vi "Delete Panel.vi"(8 "error in (no error)":errorcluster caption="错误输入（无错误）", 9 "Abort VI":bool, 10 "SelfNode*":refnum<data-value>) -> (0 "error out":errorcluster caption="错误输出", 2 "BrotherNodeBeDeleted":refnum<data-value>, 3 "ParentNode*":refnum<data-value>)   [LabVIEW 2013, in "PanelDataNode.lvclass"]
uses:
  PanelDataNode.lvclass
  PanelObject/PanelObject.lvclass
  PanelLinkNode/PanelLinkNode.lvclass/PanelLinkNode.ctl
  PanelLinkNode/PanelLinkNode.lvclass
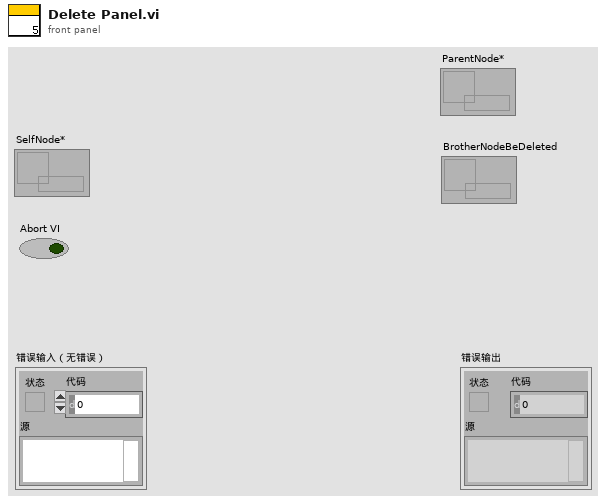
[diagram p1: front panel]
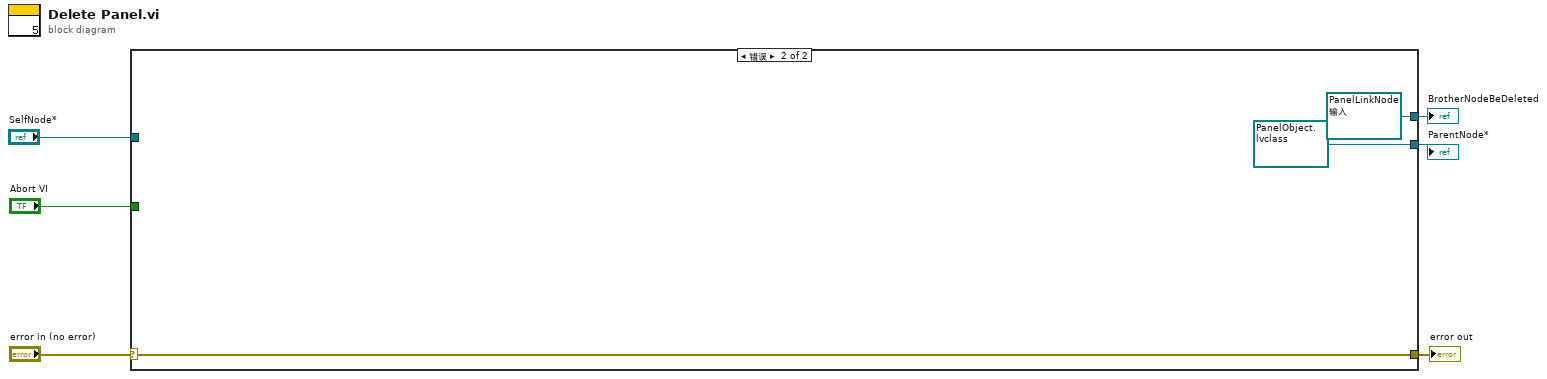
[diagram p0: block diagram]
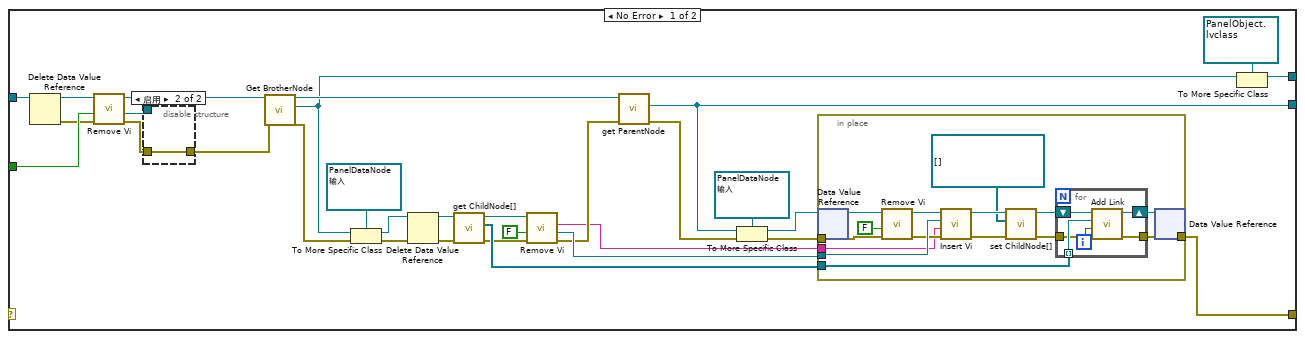
[diagram p2: hidden frame]
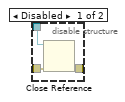
[diagram p3: hidden frame]
diagram:
  n1 = case shown="错误" "error in (no error)" {
    selector: "error in (no error)" -> [_ w65]
    tunnel: [w37 w65] -> w5
    tunnel: "SelfNode*" -> [w16 _]
    tunnel: "Abort VI" -> [w36 _]
    tunnel: [w9 refnum<data-value> refnum ("BrotherNode*")] -> w2
    tunnel: [w7 refnum<data-value> refnum ("ParentNode*")] -> w1
    frame No Error {
      n2 = Delete Data Value Reference(data value reference=w16) -> (data value=w15:refnum<class "PanelDataNode.lvclass">, error out=w14:errorcluster)  [unwired: 1 in]
      n3 = call-dynamic "Remove Vi.vi"("error in"=w14, "Abort VI"=w36, "PanelDataNode 输入"=w15) -> ("error out"=w29:errorcluster, "VI*"=w11:refnum<vi>, "PanelDataNode 输出"=w33:refnum<class "PanelDataNode.lvclass">)  [unwired: 5 in, 1 out]
      n4 = disable-structure shown="启用" {
        disable-tunnel: w29 -> [w40 w41]
        disable-tunnel: [w39 w41] -> w12
        disable-tunnel: w11 -> [w38 _]
        frame Disabled {
          n5 = Close Reference(reference=w38, error in (no error)=w40) -> (error out=w39:errorcluster)
        }
        frame Enabled {
        }
      }
      n6 = call-dynamic "Get BrotherNode.vi"("error in (no error)"=w12, "PanelLinkNode 输入"=w33) -> ("error out"=w28:errorcluster, "BrotherNode*"=w10:refnum<data-value>, "PanelLinkNode 输出"=w31:refnum<class "PanelDataNode.lvclass">)  [unwired: 7 in]
      n7 = To More Specific Class(target class=refnum<data-value> refnum ("SelfNode*"), reference=w10, error in=w28) -> (specific class reference=w21:refnum<data-value>, error out=w19:errorcluster)
      n8 = Delete Data Value Reference(data value reference=w21, error in=w19) -> (data value=w20:refnum<class "PanelDataNode.lvclass">, error out=w18:errorcluster)
      n9 = call "get ChildNode[].vi"("error in (no error)"=w18, "PanelLinkNode输入"=w20) -> ("error out"=w23:errorcluster, "ChildNode*[]"=w25:refnum<data-value>[], "PanelLinkNode输出"=w24:refnum<class "PanelDataNode.lvclass">)  [unwired: 7 in]
      n10 = call-dynamic "Remove Vi.vi"("error in"=w23, "Abort VI"=FALSE, "PanelDataNode 输入"=w24) -> ("error out"=w17:errorcluster, "VI*"=w30:refnum<vi>, "ViValue"=w13:string)  [unwired: 5 in, 1 out]
      n11 = call "get ParentNode.vi"("error in (no error)"=w17, "PanelLinkNode输入"=w31) -> ("error out"=w27:errorcluster, "ParentNode*"=w7:refnum<data-value>)  [unwired: 7 in, 1 out]
      n12 = To More Specific Class(target class=refnum<data-value> refnum ("SelfNode*"), reference=w7, error in=w27) -> (specific class reference=w34:refnum<data-value>, error out=w26:errorcluster)
      n13 = in-place {
        in-place-border: w30 -> [w54]
        in-place-border: w26 -> [w52]
        in-place-border: [w48] -> w37
        in-place-border: w25 -> [w49]
        in-place-border: w13 -> [w42]
        n14 = in-place-dvr #1(w34) -> (w56:refnum<class "PanelDataNode.lvclass">)  [unwired: 1 out]
        n15 = call-dynamic "Remove Vi.vi"("error in"=w52, "Abort VI"=FALSE, "PanelDataNode 输入"=w56) -> ("error out"=w53:errorcluster, "PanelDataNode 输出"=w55:refnum<class "PanelDataNode.lvclass">)  [unwired: 5 in, 2 out]
        n16 = call-dynamic "Insert Vi.vi"("error in (no error)"=w53, "ViValue"=w42, "VI*"=w54, "PanelDataNode 输入"=w55) -> ("error out"=w45:errorcluster, "PanelDataNode 输出"=w47:refnum<class "PanelDataNode.lvclass">)  [unwired: 6 in]
        n17 = call "set ChildNode[].vi"("error in (no error)"=w45, "ChildNode*[]"=refnum<data-value>[] [], "PanelLinkNode输入"=w47) -> ("error out"=w44:errorcluster, "PanelLinkNode输出"=w46:refnum<class "PanelDataNode.lvclass">)  [unwired: 7 in]
        n18 = for {
          tunnel: w49 -> [w60] mode=indexing
          tunnel: w44 -> [w59]
          tunnel: [w58] -> w48
          shift-right: [w61] -> w50
          shift-left: w46 -> [w62]
          i -> [w57]
          n19 = call-dynamic "Add Link.vi"("ParentLinkNode in"=w62, "ChildNode* in"=w60, "L\\R Child"=w57, "error in (no error)"=w59) -> ("ParentLinkNode out"=w61:refnum<class "PanelDataNode.lvclass">, "error out"=w58:errorcluster)  [unwired: 5 in]
        }
        n20 = in-place-dvr #1(w50) -> ()  [unwired: 2 out]
      }
      n21 = To More Specific Class(target class=refnum<data-value> refnum ("ChildNode*"), reference=w10) -> (specific class reference=w9:refnum<data-value>)  [unwired: 1 in, 1 out]
    }
    frame Error {
    }
  }
  "error out" <- w5
  "BrotherNodeBeDeleted" <- w2
  "ParentNode*" <- w1
